vi "Decimate (single).vi"(8 "error in (no error)":errorcluster, 9 "averaging (off)":bool, 10 "decimating factor (1)":i32=1, 11 "XY-data":cluster{"X-array":dbl[], "Y-array":dbl[]}) -> (0 "error out":errorcluster, 3 "Decimated XY-data out":cluster{"X-array":dbl[], "Y-array":dbl[]} {"Y-array" format="%.2p"; "X-array" format="%.2p"})   [LabVIEW 2019, in "xy_utilities.lvlib"]
doc: "Decimates the X and Y arrays of the input <b>XY-data</b> by the <b>decimating factor</b> and the <b>averaging</b> Boolean control. \n\nWire data to the data input to determine the polymorphic instance to use or manually select the instance."
uses:
  xy_utilities.lvlib
  <vilib>/Analysis/NI_AALPro.lvlib
  <vilib>/Analysis/2dsp.llb/Decimate (single shot, DBL).vi
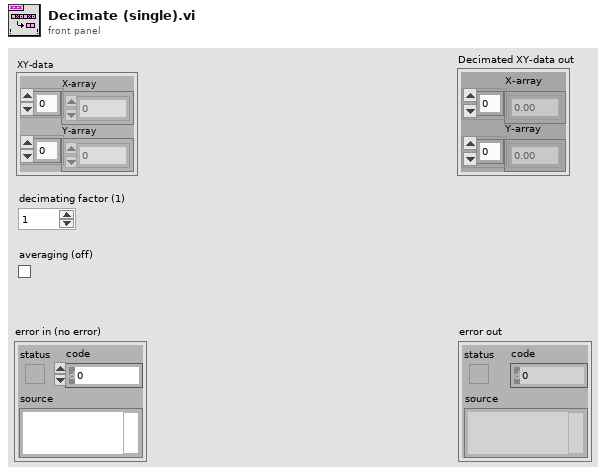
[diagram p1: front panel]
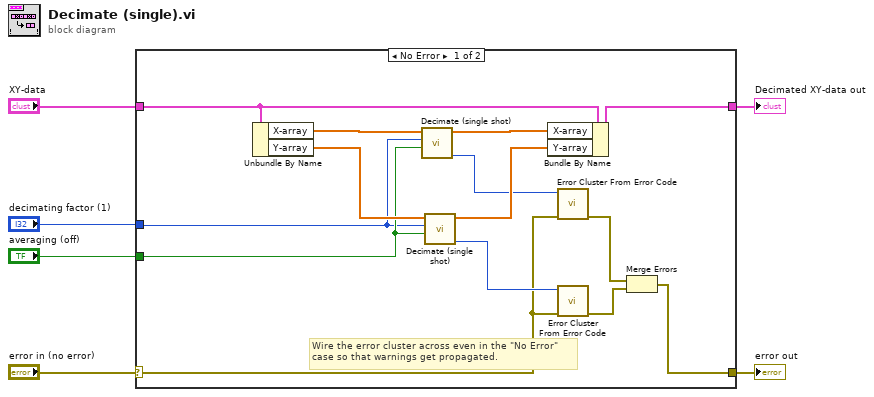
[diagram p0: block diagram]
diagram:
  n1 = case shown="No Error" "error in (no error)" {
    selector: "error in (no error)" -> [w7 w22]
    tunnel: [w8 w22] -> w5
    tunnel: "XY-data" -> [w20 w21]
    tunnel: [w19 w21] -> w3
    tunnel: "decimating factor (1)" -> [w13 _]
    tunnel: "averaging (off)" -> [w14 _]
    frame No Error {
      # "Wire the error cluster across even in the \"No Error\"\ncase so that warnings get propagated."
      n2 = Unbundle By Name(w20) -> ("X-array"=w16:dbl[], "Y-array"=w18:dbl[])
      n3 = call-poly <vilib>:"Decimate (single shot).vi"("averaging"=w14, "decimating factor"=w13, "X"=w16) -> ("error"=w9:i32, "Decimated Array"=w15:dbl[])  [unwired: 7 in]
      n4 = call-poly <vilib>:"Decimate (single shot).vi"("averaging"=w14, "decimating factor"=w13, "X"=w18) -> ("error"=w12:i32, "Decimated Array"=w17:dbl[])  [unwired: 7 in]
      n5 = Bundle By Name(cluster=w20, "X-array"=w15, "Y-array"=w17) -> (w19:cluster{"X-array":dbl[], "Y-array":dbl[]})
      n6 = call <vilib>:"Error Cluster From Error Code.vi"("error in (no error)"=w7, "error code (0)"=w9) -> ("error out"=w11:errorcluster)  [unwired: 7 in]
      n7 = call <vilib>:"Error Cluster From Error Code.vi"("error in (no error)"=w7, "error code (0)"=w12) -> ("error out"=w10:errorcluster)  [unwired: 7 in]
      n8 = Merge Errors(w11, w10) -> (w8:errorcluster)
    }
    frame Error {
    }
  }
  "error out" <- w5
  "Decimated XY-data out" <- w3
